vi "Working Example.vi"() -> ()   [LabVIEW 2020]
uses:
  pco.labview/pco.camera/Controls/binning.ctl
  pco.labview/pco.camera/Camera.lvclass
  shared/OnOffTypeDef.ctl
  pco.labview/pco.sdk/TimingControl/TimingControl.lvlib
panel:
  out "double precision float 2":dbl format="%#_17f"
  out "timestamp":T1 {"lvTimestamp" format="%<%.6X\n%x>T"}
  out "x > y?":bool
  out "Numeric":i32
  in  "Boolean":bool
  out "configuration":T3={"exposure_time_s"=nan, "delay_time_s"=nan, "roi"={"x0"=18446744073709551615, "y0"=18446744073709551615, "x1"=18446744073709551615, "y1"=18446744073709551615}, "timestamp_mode"=65535, "pixelrate"=4294967295, "trigger_mode"=65535, "acquire_mode"=65535, "metadata_mode"=65535, "noisefilter_mode"=65535, "binning"={"vert"=65535, "horz"=65535}} {"noisefilter_mode" items=["Undefined"=65535, "OFF"=0, "ON"=1]; "exposure_time_s" format="%#_6f"; "timestamp_mode" items=["Undefined"=65535, "OFF"=0, "Binary"=1, "Binary+ASCII"=2, "ASCII"=3]; "acquire_mode" items=["Undefined"=65535, "auto"=0, "external"=1, "external modulate"=2]; "trigger_mode" items=["Undefined"=65535, "auto sequence"=0, "software trigger"=1, "external exposure start & software trigger"=2, "external exposure control"=3, "external synchronized"=4, "fast external exposure control"=5, "external CDS control"=6, "slow external exposure control"=7, "external synchronized HDSDI"=258]; "metadata_mode" items=["Undefined"=65535, "OFF"=0, "ON"=1]}
  out "acq time (ms) 2":u32
  in  "Capture Now":bool
  in  "Settings.Trigger":T4
  in  "Set Trigger":bool
  out "Image":T5(plugin-control)
  out "Intensity Graph Mono":u16[][](graph)
  out "acq time (ms)":u32
  in  "Capture":bool
  in  "Init":bool
  in  "stop":bool
  out "Camera out":refnum<class "Camera.lvclass">
  out "max_height":u64
  out "max_width":u64
  out "Info Post Init":T6
  out "Info Pre Inti":T6
  in  "error in (no error)":errorcluster
  out "error out":errorcluster
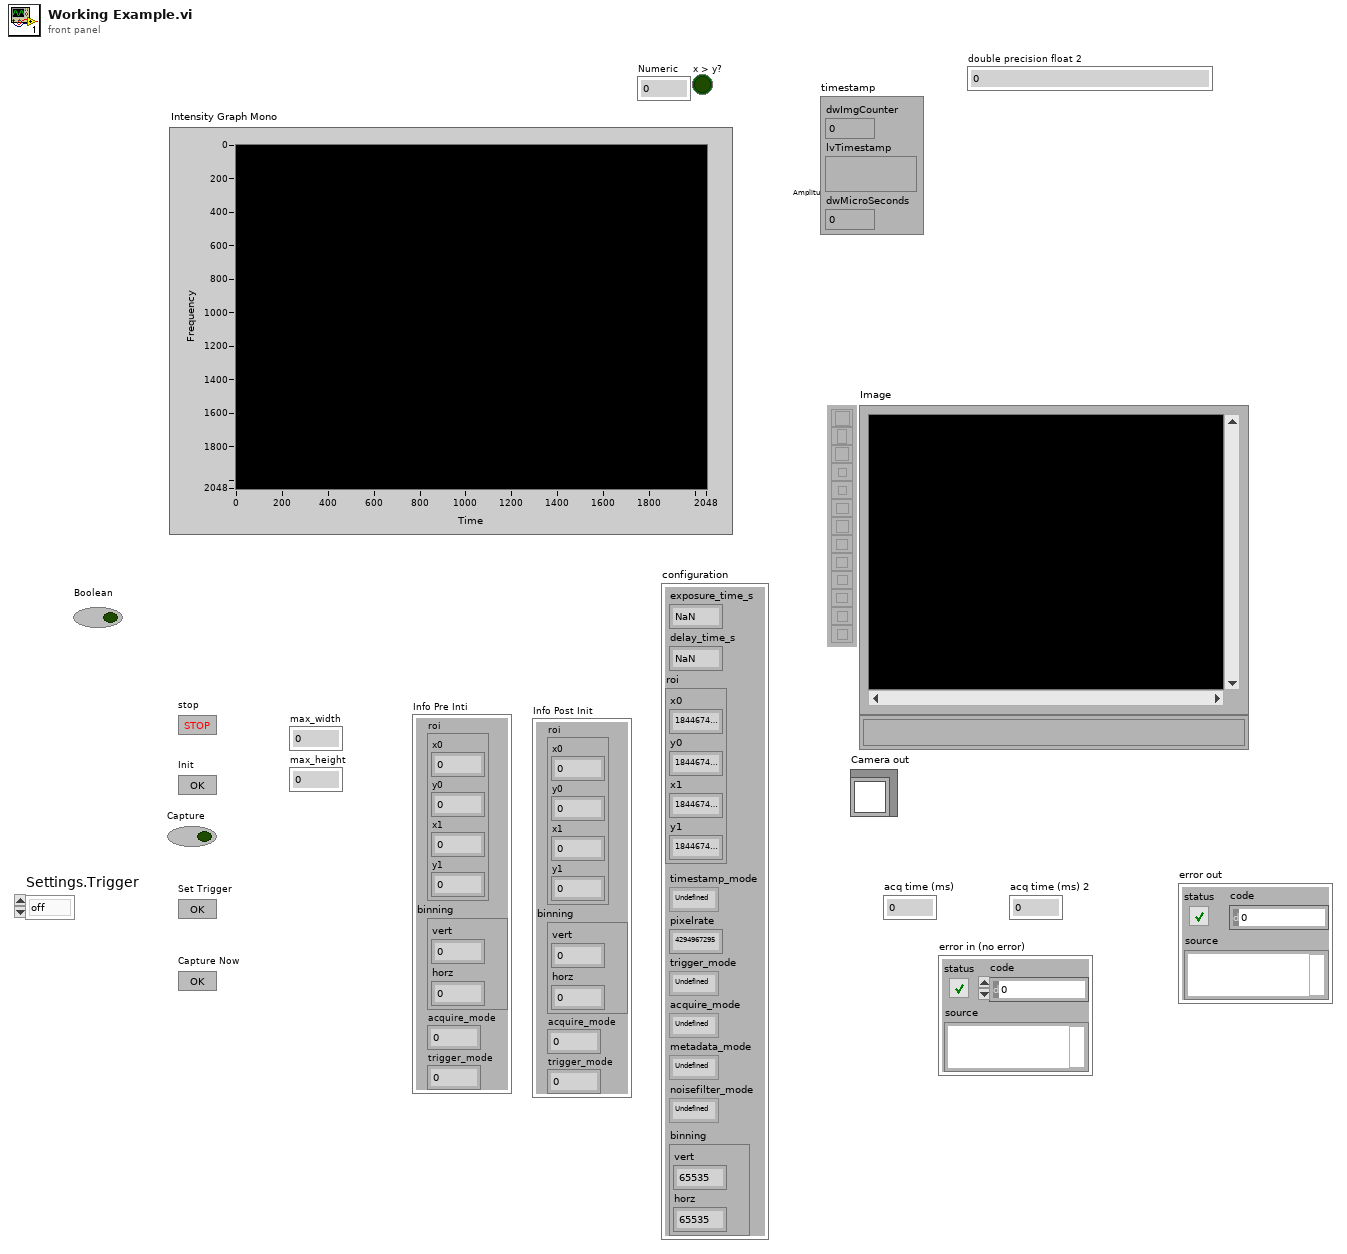
[diagram p1: front panel]
types:
  T1 = cluster{"dwImgCounter":u32, "lvTimestamp":timestamp, "dwMicroSeconds":u32}
  T2 = typedef "Camera.lvclass/binning.ctl" = cluster{"vert":u16, "horz":u16}
  T3 = cluster{"exposure_time_s":dbl, "delay_time_s":dbl, "roi":cluster{"x0":u64, "y0":u64, "x1":u64, "y1":u64}, "timestamp_mode":u16, "pixelrate":u32, "trigger_mode":u16, "acquire_mode":u16, "metadata_mode":u16, "noisefilter_mode":u16, "binning":T2}
  T4 = typedef "OnOffTypeDef.ctl" = enum16{"off", "on"}
  T5 = typedef "IMAQ Image.ctl" = refnum<image>
  T6 = cluster{"roi":cluster{"x0":u64, "y0":u64, "x1":u64, "y1":u64}, "binning":T2, "acquire_mode":u16, "trigger_mode":u16}
  T7 = enum16{"sequence", "sequence non blocking", "ring buffer", "fifo", "sequence_dpcore", "sequence_non_blocking_dpcore", "ring_buffer_dpcore", "fifo_dpcore", "tif", "multitif", "pcoraw", "b16", "dicom", "multidicom"}
  T8 = enum16{"Undefined", "Mono8", "Mono16", "BGRA8", "RGBA8", "BGRA16", "RGBA16", "CompressedMono8"}
  T9 = enum16{"auto sequence", "software trigger", "external exposure start", "external exposure control"}
  T10 = typedef "Image Type" = u32
  T11 = cluster{"serial":u32, "type":u16, "sub_type":u16, "interface_type":u16, "bit_resolution":u16, "min_exposure_time_s":dbl, "max_exposure_time_s":dbl, "min_exposure_step_s":dbl, "min_delay_time_s":dbl, "max_delay_time_s":dbl, "min_delay_step_s":dbl, "min_width":u64, "min_height":u64, "max_width":u64, "max_height":u64, "roi_step_horz":u64, "roi_step_vert":u64, "roi_symmetric_horz":bool, "roi_symmetric_vert":bool, "has_timestamp_mode":bool, "has_timestamp_mode_ascii_only":bool, "pixelrate_vec":u32[], "has_acquire_mode":bool, "has_ext_acquire_mode":bool, "has_metadata_mode":bool, "has_ram":bool, "binning_horz_vec":u16[], "binning_vert_vec":u16[]}
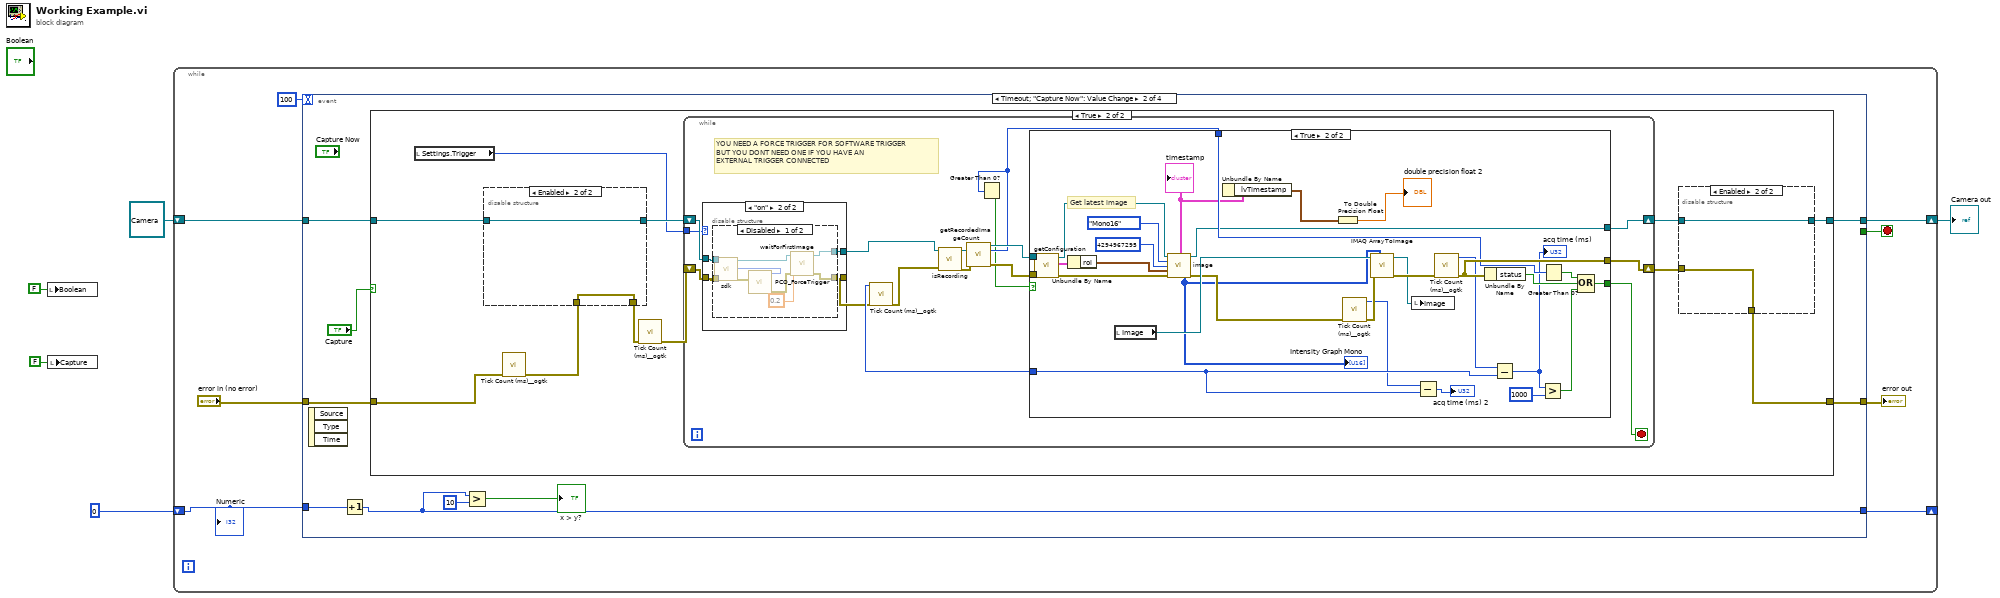
[diagram p0: block diagram]
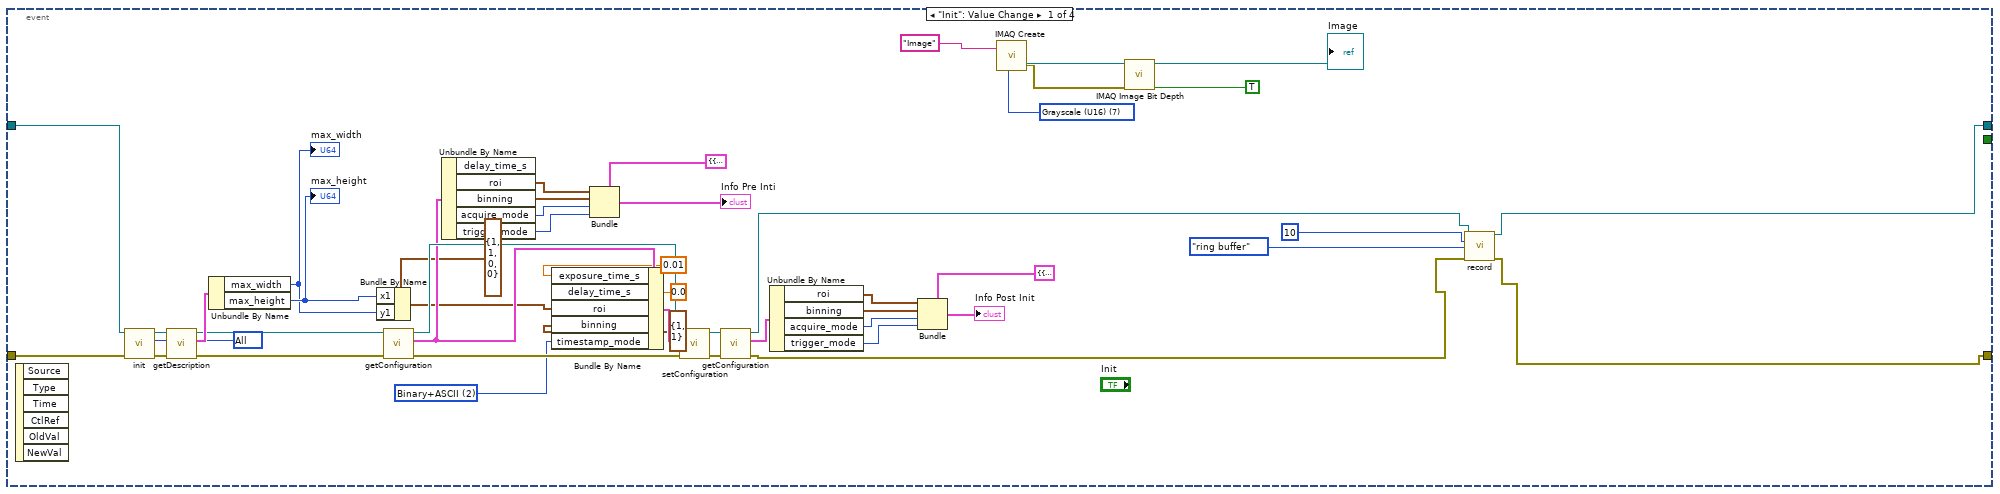
[diagram p2: hidden frame]
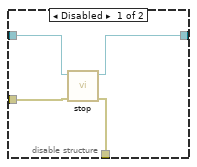
[diagram p4: hidden frame]
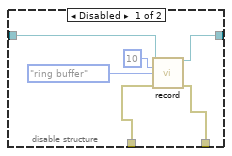
[diagram p5: hidden frame]
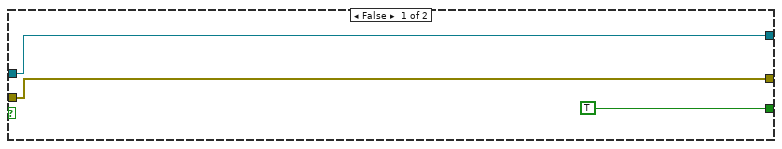
[diagram p6: hidden frame]
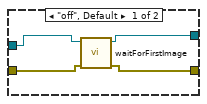
[diagram p7: hidden frame]
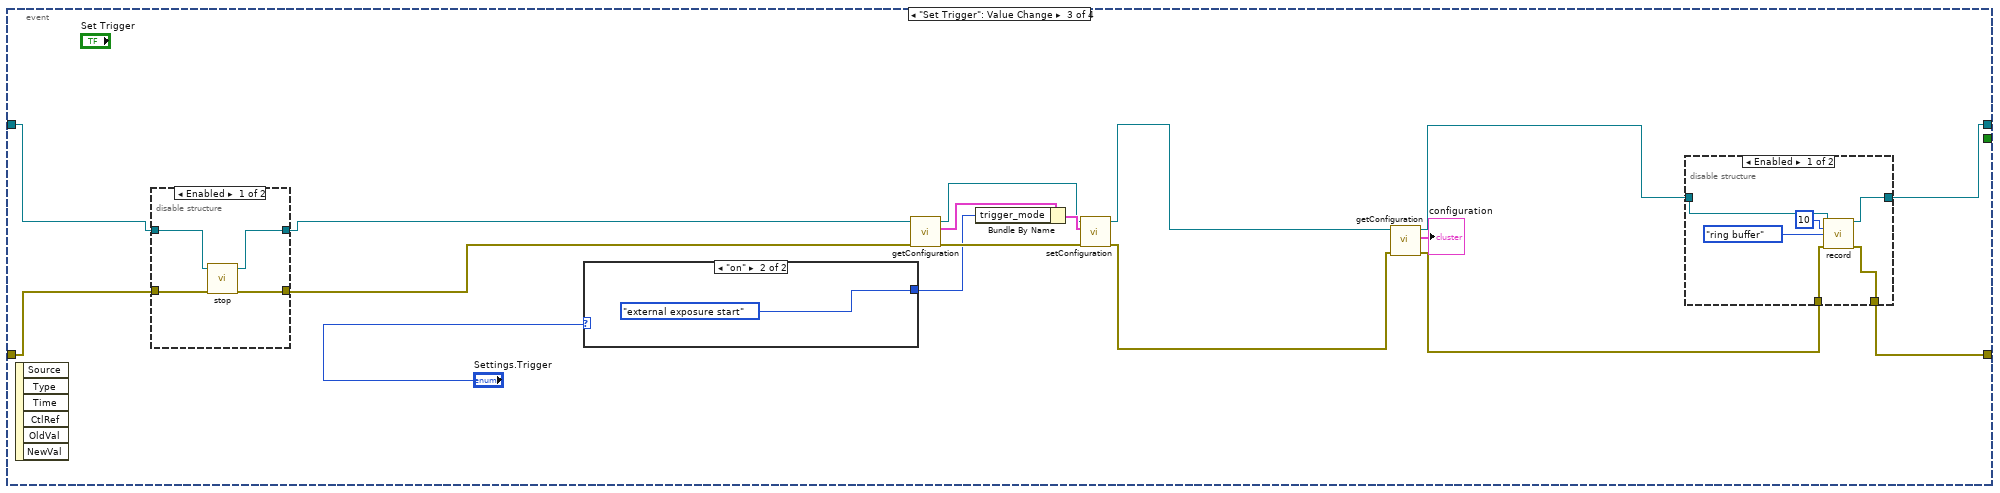
[diagram p9: hidden frame]
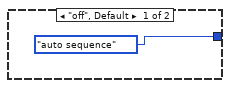
[diagram p12: hidden frame]
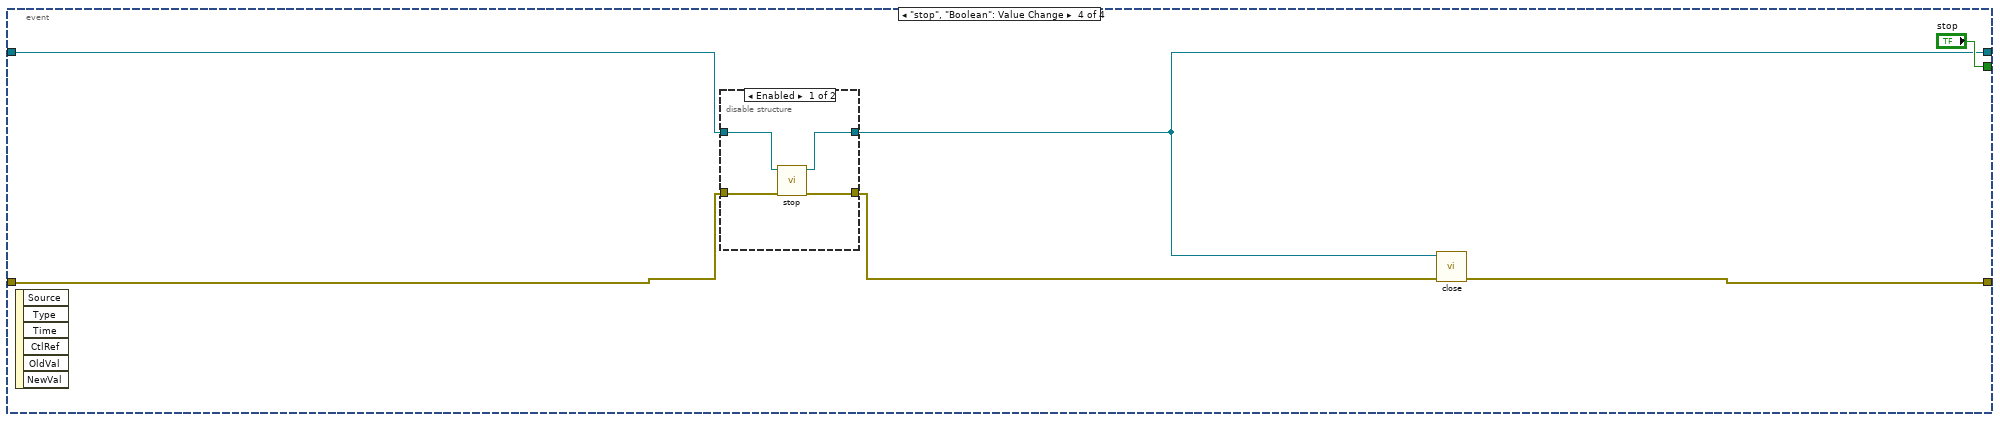
[diagram p13: hidden frame]
diagram:
  n1 = local write "Boolean"(FALSE ("Boolean")) -> ()
  n2 = local write "Capture"(FALSE ("Capture")) -> ()
  n3 = while {
    shift-right: [w10] -> w5
    shift-left: refnum<class "Camera.lvclass"> refnum ("Camera in") -> [w9]
    shift-right: [w6] -> _
    shift-left: 0 -> [w7]
    stop <- w11 stop-if-true
    n4 = event shown="[1] Timeout;  \"Capture Now\": Value Change" {
      selector: _ -> [_ _ _ _]
      dyn-events: _ -> [_ _ _ _]
      timeout: 100 -> [_ _ _ _]
      tunnel: w9 -> [w60 w69 w172 w199]
      tunnel: [w15 w68 w167 w196] -> w10
      tunnel: "error in (no error)" -> [w37 w65 w169 w198]
      tunnel: [w16 w66 w166 w200] -> w12
      tunnel: [_ _ _ "stop"] -> w11
      tunnel: w7 -> [_ w64 _ _]
      tunnel: [_ w61 _ _] -> w6
      event "Init": Value Change {
        w20 = u16 2 items=["OFF", "Binary", "Binary+ASCII", "ASCII"] ("wTimeStampMode")
        w25 = T10 7 items=["Grayscale (U8)", "Grayscale (I16)", "Grayscale (SGL)", "Complex (CSG)", "RGB (U32)", "HSL (U32)", "RGB (U64)", "Grayscale (U16)"] ("Image Type")
        w36 = u8 255 items=["FireWire"=1, "GenICam"=3, "GigE"=5, "USB"=6, "CameraLinkME4"=7, "USB3"=8, "CLHS"=11, "All"=255] ("interface")
        n5 = event-data() -> ()  [unwired: 1 in, 6 out]
        n6 = call-dynamic "init.vi"("Camera in"=w60, "interface"=w36, "error in (no error)"=w37) -> ("Camera out"=w59:refnum<class "Camera.lvclass">, "error out"=w49:errorcluster)  [unwired: 6 in]
        n7 = call-dynamic "getDescription.vi"("error in (no error)"=w49, "Camera in"=w59) -> ("error out"=w48:errorcluster, "description"=w58:T11, "Camera out"=w51:refnum<class "Camera.lvclass">)  [unwired: 7 in]
        n8 = Unbundle By Name(w58) -> ("max_width"=w30:u64, "max_height"=w31:u64)
        "max_width" <- w30
        "max_height" <- w31
        n9 = Bundle By Name(cluster=cluster{"x0":u64, "y0":u64, "x1":u64, "y1":u64} {"x0"=1, "y0"=1, "x1"=0, "y1"=0} ("roi"), "x1"=w31, "y1"=w30) -> (w29:cluster{"x0":u64, "y0":u64, "x1":u64, "y1":u64})
        n10 = call-dynamic "getConfiguration.vi"("error in (no error)"=w48, "Camera in"=w51) -> ("error out"=w47:errorcluster, "configuration"=w35:T3, "Camera out"=w50:refnum<class "Camera.lvclass">)  [unwired: 7 in]
        n11 = Unbundle By Name(w35) -> ("roi"=w57:cluster{"x0":u64, "y0":u64, "x1":u64, "y1":u64}, "binning"=w56:T2, "acquire_mode"=w55:u16, "trigger_mode"=w54:u16)  [unwired: 1 out]
        n12 = Bundle By Name(cluster=w35, "exposure_time_s"=0.01, "delay_time_s"=0.0, "roi"=w29, "binning"=T2 {"vert"=1, "horz"=1}, "timestamp_mode"=w20) -> (w34:T3)
        n13 = Bundle(cluster=T6 {"roi"={"x0"=0, "y0"=0, "x1"=0, "y1"=0}, "binning"={"vert"=0, "horz"=0}, "acquire_mode"=0, "trigger_mode"=0} ("output cluster"), "roi"=w57, "binning"=w56, "acquire_mode"=w55, "trigger_mode"=w54) -> (→"Info Pre Inti":T6)
        n14 = call-dynamic "setConfiguration.vi"("error in (no error)"=w47, "configuration"=w34, "Camera in"=w50) -> ("error out"=w43:errorcluster, "Camera out"=w44:refnum<class "Camera.lvclass">)  [unwired: 7 in]
        n15 = call-dynamic "getConfiguration.vi"("error in (no error)"=w43, "Camera in"=w44) -> ("error out"=w17:errorcluster, "configuration"=w42:T3, "Camera out"=w14:refnum<class "Camera.lvclass">)  [unwired: 7 in]
        n16 = Unbundle By Name(w42) -> ("roi"=w41:cluster{"x0":u64, "y0":u64, "x1":u64, "y1":u64}, "binning"=w40:T2, "acquire_mode"=w39:u16, "trigger_mode"=w38:u16)
        n17 = Bundle(cluster=T6 {"roi"={"x0"=0, "y0"=0, "x1"=0, "y1"=0}, "binning"={"vert"=0, "horz"=0}, "acquire_mode"=0, "trigger_mode"=0} ("output cluster"), "roi"=w41, "binning"=w40, "acquire_mode"=w39, "trigger_mode"=w38) -> (→"Info Post Init":T6)
        n18 = call "IMAQ Create"("Image Name"="Image", "Image Type"=w25) -> ("New Image"=w24:T5, "error out"=w21:errorcluster)  [unwired: 3 in]
        n19 = call "IMAQ Image Bit Depth"("Image"=w24, "error in (no error)"=w21, "Get/Set Bit Depth? (Set)"=TRUE) -> ("Image Out"=→"Image":T5)  [unwired: 10 in, 2 out]
        n20 = call-dynamic "record.vi"("Camera in"=w14, "num_images"=u32 10, "record_mode"=T7."ring buffer", "error in (no error)"=w17) -> ("Camera out"=w15:refnum<class "Camera.lvclass">, "error out"=w16:errorcluster)  [unwired: 10 in]
      }
      event Timeout; "Capture Now": Value Change {
        n21 = event-data() -> ()  [unwired: 1 in, 3 out]
        n22 = Increment(x=w64) -> (x+1=w61:i32)
        n23 = case shown="True" "Capture" {
          tunnel: w69 -> [w71 w82]
          tunnel: [w71 w79] -> w68
          tunnel: [w70 w77] -> w66
          tunnel: w65 -> [w70 w76]
          frame False {
          }
          frame True {
            n24 = local read "Settings.Trigger"() -> (w72:T4)
            n25 = call <userlib>:"Tick Count (ms)__ogtk.vi"("error in (no error)"=w76) -> ("error out"=w75:errorcluster)  [unwired: 9 in, 1 out]
            n26 = disable-structure shown="Enabled" {
              disable-tunnel: w82 -> [w94 w96]
              disable-tunnel: [w93 w96] -> w81
              disable-tunnel: w75 -> [w92 w95]
              disable-tunnel: [w91 w95] -> w74
              frame Disabled {
                n27 = call-dynamic "record.vi"("Camera in"=w94, "num_images"=u32 10, "record_mode"=T7."ring buffer", "error in (no error)"=w92) -> ("Camera out"=w93:refnum<class "Camera.lvclass">, "error out"=w91:errorcluster)  [unwired: 10 in]
              }
              frame Enabled {
              }
            }
            n28 = call <userlib>:"Tick Count (ms)__ogtk.vi"("error in (no error)"=w74) -> ("error out"=w73:errorcluster)  [unwired: 9 in, 1 out]
            n29 = while {
              tunnel: w72 -> [w104]
              shift-right: [w109] -> w80
              shift-left: w81 -> [w110]
              shift-right: [w108] -> w78
              shift-left: w73 -> [w105]
              stop <- w99 stop-if-true
              # "YOU NEED A FORCE TRIGGER FOR SOFTWARE TRIGGER \nBUT YOU DONT NEED ONE IF YOU HAVE AN \nEXTERNAL TRIGGER CONNECTED"
              n30 = case shown="\"on\"" w104 {
                tunnel: [w146 w150] -> w107
                tunnel: [w148 w151] -> w111
                tunnel: w105 -> [w147 w153]
                tunnel: w110 -> [w149 w152]
                frame "off", Default {
                  n31 = call-dynamic "waitForFirstImage.vi"("error in (no error)"=w147, "Camera in"=w149) -> ("error out"=w146:errorcluster, "Camera out"=w148:refnum<class "Camera.lvclass">)  [unwired: 8 in]
                }
                frame "on" {
                  n32 = disable-structure shown="Disabled" {
                    disable-tunnel: w153 -> [w160 w163]
                    disable-tunnel: w152 -> [w159 w164]
                    disable-tunnel: [w158 w164] -> w151
                    disable-tunnel: [w155 w163] -> w150
                    frame Disabled {
                      n33 = call-dynamic "sdk.vi"("Camera in"=w159, "error in (no error)"=w160) -> ("Camera out"=w157:refnum<class "Camera.lvclass">, "sdk"=w161:u64, "error out"=w162:errorcluster)  [unwired: 11 in]
                      n34 = call "PCO_ForceTrigger.vi"("error in (no error)"=w162, "ph"=w161) -> ("error out"=w156:errorcluster)  [unwired: 6 in, 3 out]
                      n35 = call-dynamic "waitForFirstImage.vi"("error in (no error)"=w156, "timeout_s"=0.2, "Camera in"=w157) -> ("error out"=w155:errorcluster, "Camera out"=w158:refnum<class "Camera.lvclass">)  [unwired: 7 in]
                    }
                    frame Enabled {
                    }
                  }
                }
              }
              n36 = call <userlib>:"Tick Count (ms)__ogtk.vi"("error in (no error)"=w107) -> ("error out"=w106:errorcluster, "millisecond timer value"=w112:u32)  [unwired: 9 in]
              n37 = call-dynamic "isRecording.vi"("Camera in"=w111, "error in (no error)"=w106) -> ("Camera out"=w101:refnum<class "Camera.lvclass">, "error out"=w100:errorcluster)  [unwired: 11 in, 1 out]
              n38 = call-dynamic "getRecordedImageCount.vi"("Camera in"=w101, "error in (no error)"=w100) -> ("Camera out"=w103:refnum<class "Camera.lvclass">, "recorded_image_count"=w98:u32, "error out"=w102:errorcluster)  [unwired: 11 in]
              n39 = Greater Than 0?(x=w98) -> (x > 0?=w97:bool)
              n40 = case shown="True" w97 {
                tunnel: w112 -> [_ w145]
                tunnel: [w115 w119] -> w109
                tunnel: [w114 w144] -> w108
                tunnel: w103 -> [w115 w138]
                tunnel: w98 -> [_ w133]
                tunnel: w102 -> [w114 w130]
                tunnel: [TRUE w121] -> w99
                frame False {
                }
                frame True {
                  # "Get latest image"
                  n41 = call-dynamic "getConfiguration.vi"("error in (no error)"=w130, "Camera in"=w138) -> ("error out"=w129:errorcluster, "configuration"=w141:T3, "Camera out"=w139:refnum<class "Camera.lvclass">)  [unwired: 7 in]
                  n42 = Unbundle By Name(w141) -> ("roi"=w140:cluster{"x0":u64, "y0":u64, "x1":u64, "y1":u64})
                  n43 = local read "Image"() -> (w127:T5)
                  n44 = call-dynamic "image.vi"("Camera in"=w139, "data_format"=T8."Mono16", "image_index"=u32 4294967295 ("dwImgIdx"), "roi"=w140, "error in (no error)"=w129) -> ("timestamp"=w118:T1, "Camera out"=w119:refnum<class "Camera.lvclass">, "raw_image (U16)"=w120:u16[][], "error out"=w125:errorcluster)  [unwired: 3 in, 4 out]
                  "Intensity Graph Mono" <- w120
                  "timestamp" <- w118
                  n45 = Unbundle By Name(w118) -> ("lvTimestamp"=w117:timestamp)
                  n46 = To Double Precision Float(number=w117) -> (double precision float=→"double precision float 2":dbl)
                  n47 = call <userlib>:"Tick Count (ms)__ogtk.vi"("error in (no error)"=w125) -> ("error out"=w124:errorcluster, "millisecond timer value"=w123:u32)  [unwired: 9 in]
                  n48 = call "IMAQ ArrayToImage"("Image Pixels (U16)"=w120, "error in (no error)"=w124, "Image"=w127) -> ("error out"=w137:errorcluster, "Image Out"=w126:T5)  [unwired: 7 in]
                  n49 = local write "Image"(w126) -> ()
                  n50 = Subtract(x=w123, y=w145) -> (x-y=→"acq time (ms) 2":u32)
                  n51 = call <userlib>:"Tick Count (ms)__ogtk.vi"("error in (no error)"=w137) -> ("error out"=w144:errorcluster, "millisecond timer value"=w136:u32)  [unwired: 9 in]
                  n52 = Unbundle By Name(w144) -> ("status"=w134:bool)
                  n53 = Subtract(x=w136, y=w145) -> (x-y=w131:u32)
                  "acq time (ms)" <- w131
                  n54 = Greater?(x=w131, y=u32 1000) -> (0:w135:bool)
                  n55 = Greater Than 0?(x=w133) -> (x > 0?=w132:bool)
                  n56 = Compound Arithmetic op=OR(w132, w134, w135) -> (w121:bool)
                }
              }
            }
            n57 = disable-structure shown="Enabled" {
              disable-tunnel: w80 -> [w86 w87]
              disable-tunnel: [w85 w87] -> w79
              disable-tunnel: w78 -> [w84 w88]
              disable-tunnel: [w83 w88] -> w77
              frame Disabled {
                n58 = call-dynamic "stop.vi"("error in (no error)"=w84, "Camera in"=w86) -> ("error out"=w83:errorcluster, "Camera out"=w85:refnum<class "Camera.lvclass">)  [unwired: 8 in]
              }
              frame Enabled {
              }
            }
          }
        }
        n59 = Greater?(x=w61, y=10) -> (0:→"x > y?":bool)
      }
      event "Set Trigger": Value Change {
        n60 = event-data() -> ()  [unwired: 1 in, 6 out]
        n61 = disable-structure shown="Enabled" {
          disable-tunnel: w172 -> [w191 w193]
          disable-tunnel: [w190 w193] -> w171
          disable-tunnel: [w189 w192] -> w170
          disable-tunnel: w169 -> [w188 w192]
          frame Enabled {
            n62 = call-dynamic "stop.vi"("error in (no error)"=w188, "Camera in"=w191) -> ("error out"=w189:errorcluster, "Camera out"=w190:refnum<class "Camera.lvclass">)  [unwired: 8 in]
          }
          frame Disabled {
          }
        }
        n63 = case shown="\"on\"" "Settings.Trigger" {
          tunnel: [T9."auto sequence" ("TriggerMode") T9."external exposure start" ("TriggerMode")] -> w179
          frame "off", Default {
          }
          frame "on" {
          }
        }
        n64 = call-dynamic "getConfiguration.vi"("error in (no error)"=w170, "Camera in"=w171) -> ("error out"=w181:errorcluster, "configuration"=w178:T3, "Camera out"=w177:refnum<class "Camera.lvclass">)  [unwired: 7 in]
        n65 = Bundle By Name(cluster=w178, "trigger_mode"=w179) -> (w180:T3)
        n66 = call-dynamic "setConfiguration.vi"("error in (no error)"=w181, "configuration"=w180, "Camera in"=w177) -> ("error out"=w173:errorcluster, "Camera out"=w175:refnum<class "Camera.lvclass">)  [unwired: 7 in]
        n67 = call-dynamic "getConfiguration.vi"("error in (no error)"=w173, "Camera in"=w175) -> ("error out"=w165:errorcluster, "configuration"=→"configuration":T3, "Camera out"=w168:refnum<class "Camera.lvclass">)  [unwired: 7 in]
        n68 = disable-structure shown="Enabled" {
          disable-tunnel: [w187 _] -> w167
          disable-tunnel: [w186 _] -> w166
          disable-tunnel: w168 -> [w183 _]
          disable-tunnel: w165 -> [w182 _]
          frame Enabled {
            n69 = call-dynamic "record.vi"("Camera in"=w183, "num_images"=u32 10, "record_mode"=T7."ring buffer", "error in (no error)"=w182) -> ("Camera out"=w187:refnum<class "Camera.lvclass">, "error out"=w186:errorcluster)  [unwired: 10 in]
          }
          frame Disabled {
          }
        }
      }
      event "stop", "Boolean": Value Change {
        n70 = event-data() -> ()  [unwired: 1 in, 6 out]
        n71 = disable-structure shown="Enabled" {
          disable-tunnel: w199 -> [w205 w207]
          disable-tunnel: [w204 w207] -> w196
          disable-tunnel: [w203 w206] -> w197
          disable-tunnel: w198 -> [w202 w206]
          frame Enabled {
            n72 = call-dynamic "stop.vi"("error in (no error)"=w202, "Camera in"=w205) -> ("error out"=w203:errorcluster, "Camera out"=w204:refnum<class "Camera.lvclass">)  [unwired: 8 in]
          }
          frame Disabled {
          }
        }
        n73 = call-dynamic "close.vi"("error in (no error)"=w197, "Camera in"=w196) -> ("error out"=w200:errorcluster)  [unwired: 9 in]
      }
    }
    "error out" <- w12
    "Numeric" <- w7
  }
  "Camera out" <- w5
